vi "main.vi"() -> ()   [LabVIEW 2022 SP3]
uses:
  State_control.ctl
  <vilib>/Instr/_visa.llb/VISA Configure Serial Port (Instr).vi
panel:
  out "Waveform Chart":dbl(graph)
  in  "Stop":bool
  in  "Start meas":bool
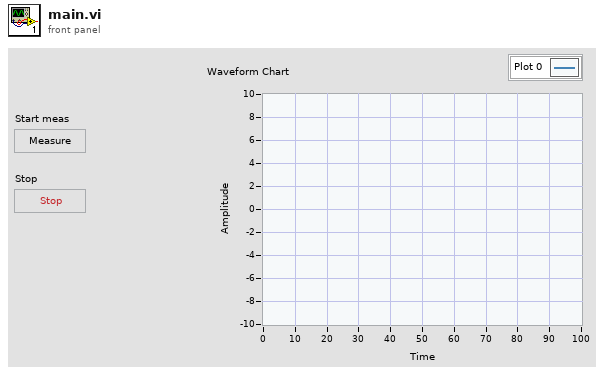
[diagram p1: front panel]
types:
  T1 = typedef "State_control.ctl" = enum16{"Init", "Waiting", "Measure", "Finish"}
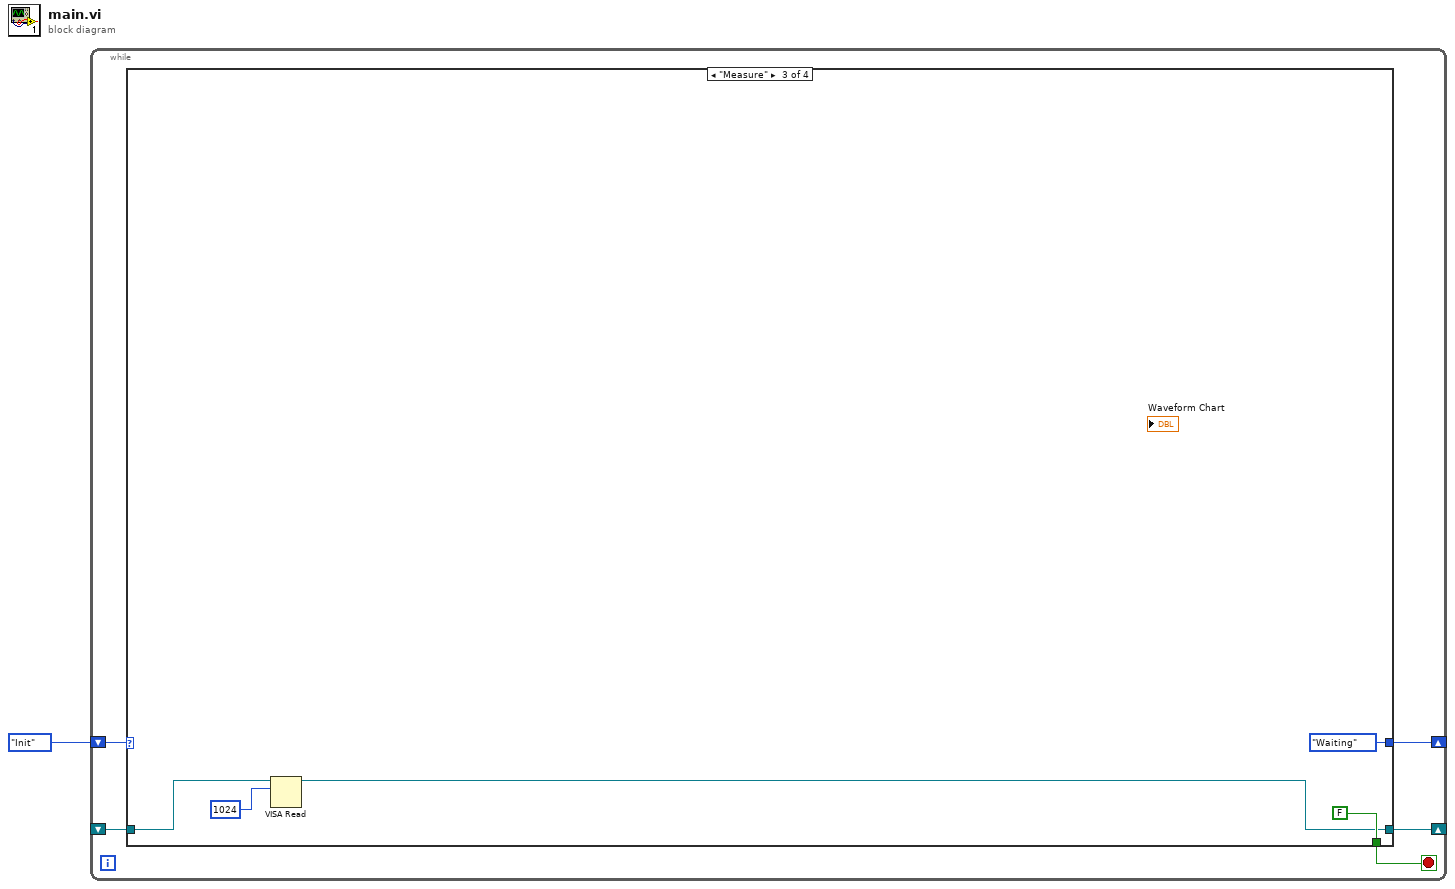
[diagram p0: block diagram]
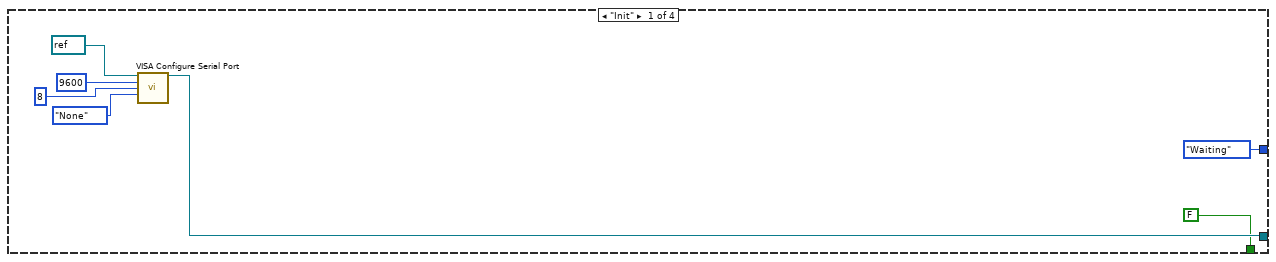
[diagram p2: hidden frame]
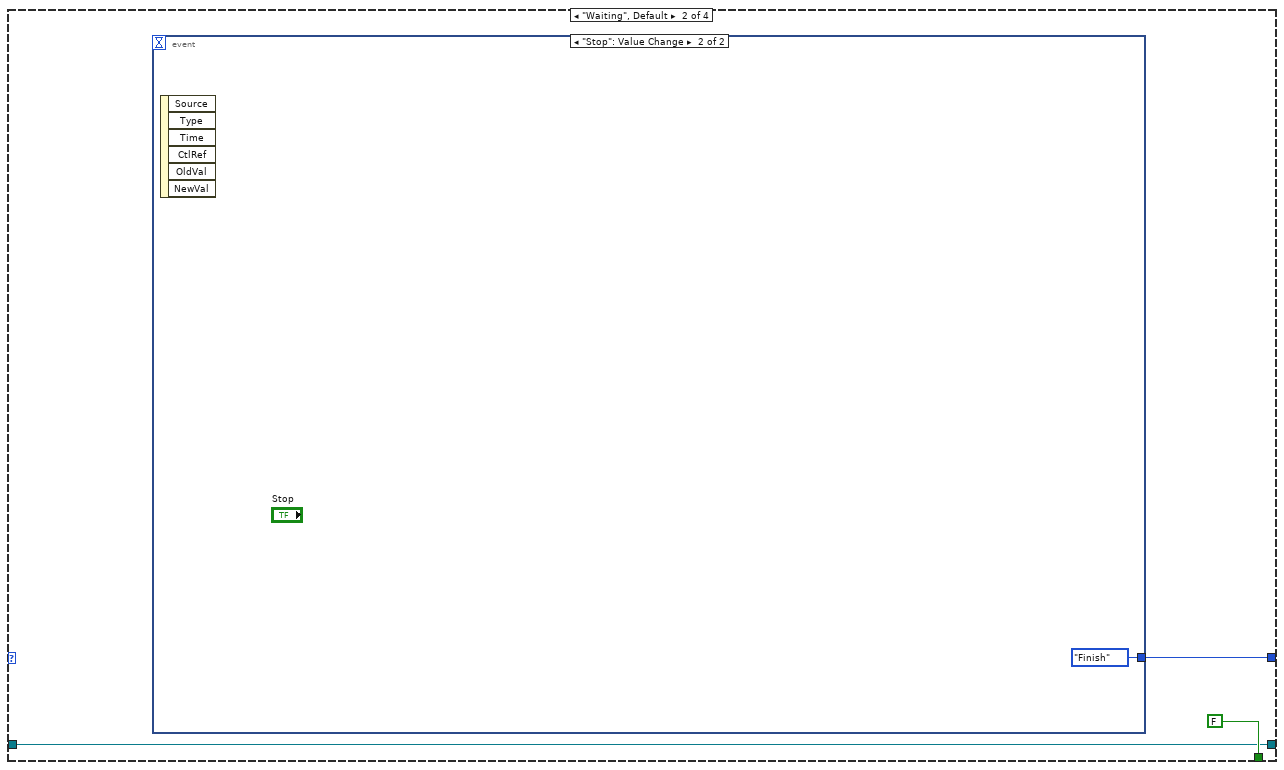
[diagram p3: hidden frame]
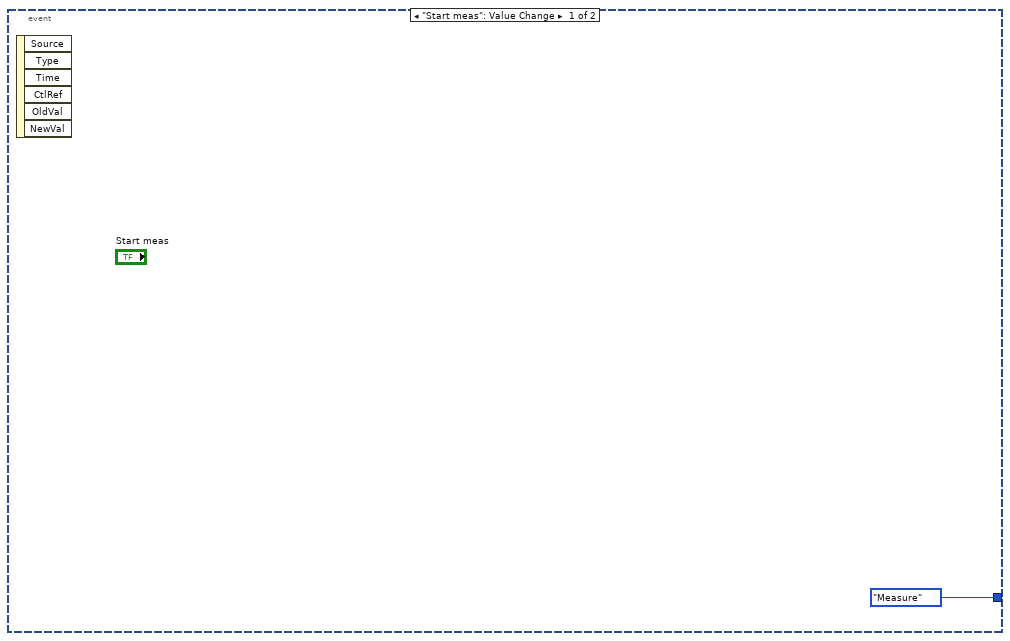
[diagram p4: hidden frame]
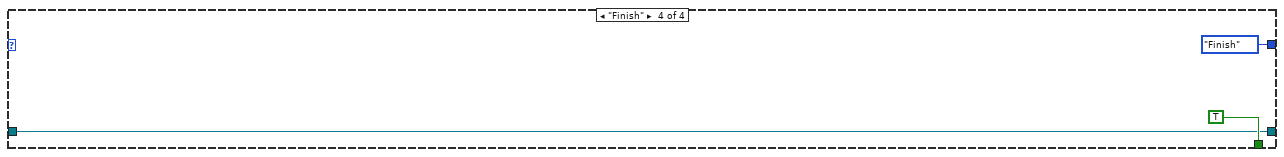
[diagram p5: hidden frame]
diagram:
  n1 = while {
    shift-right: [w3] -> _
    shift-left: State_control."Init" ("State") -> [w6]
    shift-right: [w5] -> _
    shift-left: _ -> [w4]
    stop <- w2 stop-if-true
    n2 = case shown="\"Measure\"" w6 {
      tunnel: [w9 w14 w20 w24] -> w5
      tunnel: w4 -> [_ w14 w23 w24]
      tunnel: [State_control."Waiting" ("State 2") w16 State_control."Waiting" ("State 2") State_control."Finish" ("State 2")] -> w3
      tunnel: [FALSE FALSE FALSE TRUE] -> w2
      frame "Init" {
        n3 = call-poly "VISA Configure Serial Port"("VISA resource name"=refnum<visa-resource-name> refnum, "baud rate (9600)"=u32 9600, "data bits (8)"=u16 8, "parity (0:none)"=enum16{"None", "Odd", "Even", "Mark", "Space"}."None") -> ("VISA resource name out"=w9:refnum<visa-resource-name>)  [unwired: 10 in, 1 out]
      }
      frame "Waiting", Default {
        n4 = event shown="[1] \"Stop\": Value Change" {
          selector: _ -> [_ _]
          dyn-events: _ -> [_ _]
          timeout: _ -> [_ _]
          tunnel: [State_control."Measure" ("State 2") State_control."Finish" ("State 2")] -> w16
          event "Start meas": Value Change {
            n5 = event-data() -> ()  [unwired: 1 in, 6 out]
          }
          event "Stop": Value Change {
            n6 = event-data() -> ()  [unwired: 1 in, 6 out]
          }
        }
      }
      frame "Measure" {
        n7 = VISA Read(VISA resource name=w23, byte count=u32 1024) -> (VISA resource name out=w20:refnum<visa-resource-name>)  [unwired: 1 in, 3 out]
      }
      frame "Finish" {
      }
    }
  }
